vi "sharpdeadzone.vi"(1 "Size":i16, 2 "in":i16) -> (0 "out":i16)   [LabVIEW 2010, in "Wall Follower.lvrbt"]
uses:
  Wall Follower.lvrbt
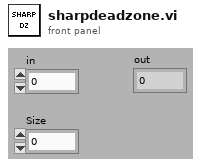
[diagram p1: front panel]
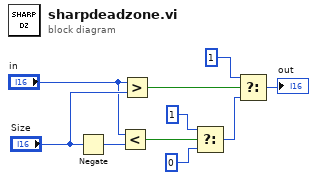
[diagram p0: block diagram]
diagram:
  n1 = Negate(x="Size") -> (-x=w5:i16)
  n2 = Less?(x="in", y=w5) -> (x < y?=w3:bool)
  n3 = Greater?(x="in", y="Size") -> (0:w9:bool)
  n4 = Select(t=i16 1, s=w3, f=i16 0) -> (s? t:f=w7:i16)
  n5 = Select(t=i16 1, s=w9, f=w7) -> (s? t:f=→"out":i16)
